vi "Construct Header Data Packet Return.vi"(11 "Packet Return":refnum<class "IPacket Return.lvclass">) -> (3 "Header Data Packet Return out":refnum<class "Header Data Packet Return.lvclass">)   [LabVIEW 2020, in "Network Messenger.lvlib" / "Header Data Packet Return.lvclass"]
uses:
  <vilib>/gpm_packages/@cs/Network-interface/Source/Network Messenger/Header Data Packet Return/Header Data Packet Return.lvclass
  <vilib>/gpm_packages/@cs/Network-interface/Source/Network Messenger/IPacket Return/IPacket Return.lvclass
  <vilib>/gpm_packages/@cs/Network-interface/Source/Network Messenger/Header Data Packet Return/Header Data Packet Return.lvclass/Header Data Packet Return.ctl
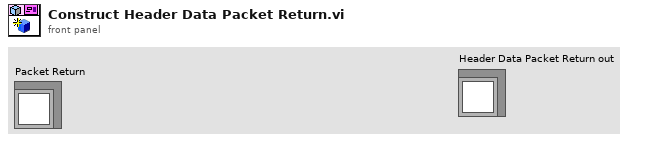
[diagram p1: front panel]
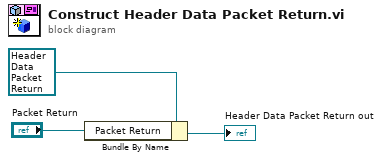
[diagram p0: block diagram]
diagram:
  n1 = Bundle By Name(cluster=refnum<class "Header Data Packet Return.lvclass"> refnum ("Header Data Packet Return in"), "Packet Return"="Packet Return") -> (→"Header Data Packet Return out":refnum<class "Header Data Packet Return.lvclass">)
